vi "RectConvert.vi"(11 "rect":T3 caption="矩形") -> (2 "RectWH":T1, 3 "RectTB":T2)   [LabVIEW 2012, in "Picture Box Tools.lvlib"]
uses:
  Picture Box Tools.lvlib
  RectTB/RectTB.ctl
  RectWH/RectWH.ctl
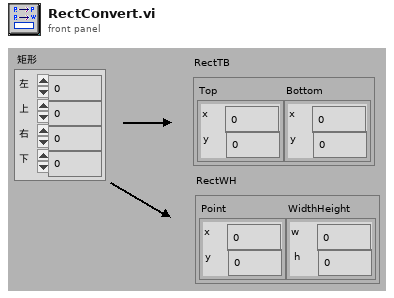
[diagram p1: front panel]
types:
  T1 = typedef "Picture Box Tools.lvlib/RectWH.ctl" = cluster{"Point":cluster{"x":i16, "y":i16}, "WidthHeight":cluster{"x":i16, "y":i16}}
  T2 = typedef "Picture Box Tools.lvlib/RectTB.ctl" = cluster{"Top":cluster{"x":i16, "y":i16}, "Bottom":cluster{"x":i16, "y":i16}}
  T3 = cluster{"left":i16, "top":i16, "right":i16, "bottom":i16}
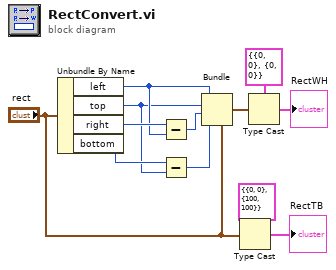
[diagram p0: block diagram]
diagram:
  n1 = Unbundle By Name("rect") -> ("left"=w9:i16, "top"=w8:i16, "right"=w11:i16, "bottom"=w10:i16)
  n2 = Subtract(x=w11, y=w9) -> (x-y=w7:i16)
  n3 = Subtract(x=w10, y=w8) -> (x-y=w6:i16)
  n4 = Bundle(cluster="rect", "left"=w9, "top"=w8, "right"=w7, "bottom"=w6) -> (w5:T3)
  n5 = Type Cast(type=T2 {"Top"={"x"=0, "y"=0}, "Bottom"={"x"=100, "y"=100}} ("RectTB"), x="rect") -> (*(type *) &x=→"RectTB":T2)
  n6 = Type Cast(type=T1 {"Point"={"x"=0, "y"=0}, "WidthHeight"={"x"=0, "y"=0}} ("RectWH"), x=w5) -> (*(type *) &x=→"RectWH":T1)
